vi "startScanManual.vi"(8 "error in (no error)":errorcluster, 11 "ElectrometerController in":refnum<class "ElectrometerController.lvclass">) -> (0 "error out":errorcluster, 3 "ElectrometerController out":refnum<class "ElectrometerController.lvclass">)   [LabVIEW 2016, in "ElectrometerController.lvclass"]
uses:
  ElectrometerController.lvclass
  Electrometer/State/ElectrometerState.lvclass
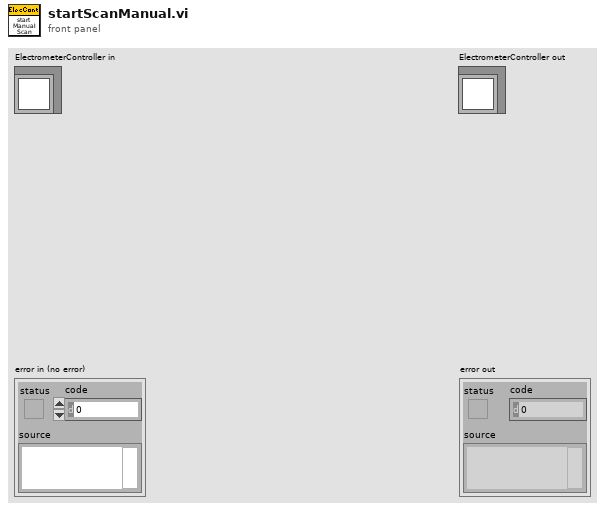
[diagram p1: front panel]
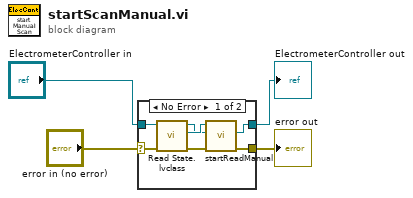
[diagram p0: block diagram]
diagram:
  n1 = case shown="No Error" "error in (no error)" {
    selector: "error in (no error)" -> [w6 w13]
    tunnel: [w8 w13] -> w3
    tunnel: [w9 w12] -> w1
    tunnel: "ElectrometerController in" -> [w7 w12]
    frame No Error {
      n2 = call-dynamic "Read State.lvclass.vi"("error in (no error)"=w6, "ElectrometerController in"=w7) -> ("error out"=w5:errorcluster, "ElectrometerState"=w11:refnum<class "ElectrometerState.lvclass">, "ElectrometerController out"=w10:refnum<class "ElectrometerController.lvclass">)  [unwired: 7 in]
      n3 = call-dynamic "startReadManual.vi"("error in (no error)"=w5, "ElectrometerController in"=w10, "State in"=w11) -> ("error out"=w8:errorcluster, "ElectrometerController. out"=w9:refnum<class "ElectrometerController.lvclass">)  [unwired: 6 in, 1 out]
    }
    frame Error {
    }
  }
  "error out" <- w3
  "ElectrometerController out" <- w1
